vi "Write Robot Speed Limit.vi"(8 "error in":errorcluster, 10 "Speed Limit":refnum<class "Vec3d Class.lvclass">, 11 "Gantry in":refnum<class "Gantry Class.lvclass">) -> (0 "error out":errorcluster, 3 "Gantry out":refnum<class "Gantry Class.lvclass">)   [LabVIEW 2011, in "Gantry Class.lvclass"]
uses:
  Gantry Class.lvclass
  Vec3d Class/Vec3d Class.lvclass
  Gantry Class.lvclass/Gantry Class.ctl
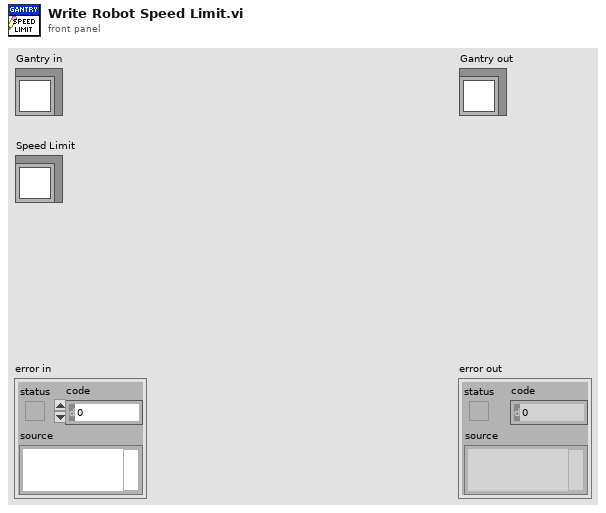
[diagram p1: front panel]
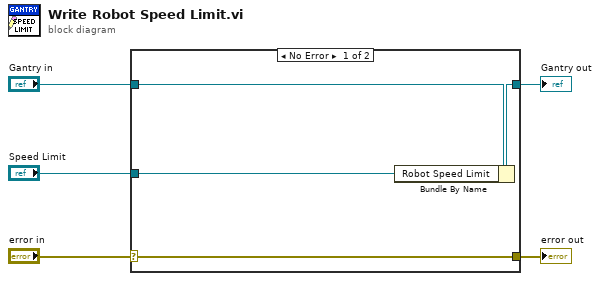
[diagram p0: block diagram]
diagram:
  n1 = case shown="No Error" "error in" {
    selector: "error in" -> [w9 w10]
    tunnel: [w9 w10] -> w4
    tunnel: [w7 w11] -> w2
    tunnel: "Gantry in" -> [w8 w11]
    tunnel: "Speed Limit" -> [w6 _]
    frame No Error {
      n2 = Bundle By Name(cluster=w8, "Robot Speed Limit"=w6) -> (w7:refnum<class "Gantry Class.lvclass">)
    }
    frame Error {
    }
  }
  "error out" <- w4
  "Gantry out" <- w2
